vi "Parse Data Object Simple.vi"(11 "Data":T1(array[cluster])) -> (0 "ROI 1, Frame 1, Row 1":dbl[](graph), 3 "ROI 1, Frame 1":dbl[][](graph))   [LabVIEW 2015, in "LightField Automation.lvclass"]
uses:
  LightField Automation.lvclass
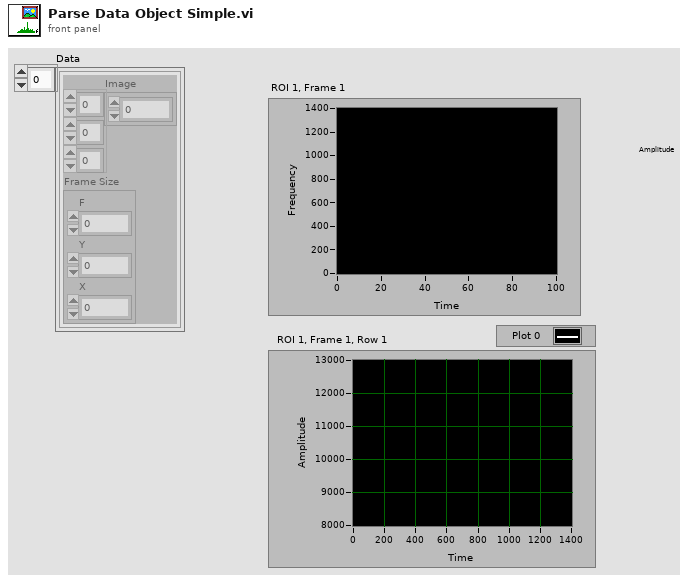
[diagram p1: front panel]
types:
  T1 = cluster{"Image":dbl[][][], "Frame Size":cluster{"F":i32, "Y":i32, "X":i32}}[]
  T2 = cluster{"Image":dbl[][][], "Frame Size":cluster{"F":i32, "Y":i32, "X":i32}}
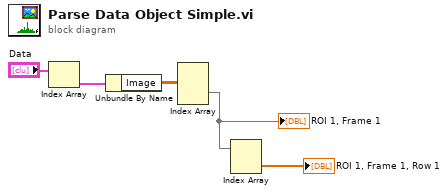
[diagram p0: block diagram]
diagram:
  n1 = Index Array(array="Data") -> (element=w5:T2)  [unwired: 1 in]
  n2 = Unbundle By Name(w5) -> ("Image"=w4:dbl[][][])
  n3 = Index Array(array=w4) -> (element=w3:dbl[][])  [unwired: 3 in]
  "ROI 1, Frame 1" <- w3
  n4 = Index Array(array=w3) -> (element=→"ROI 1, Frame 1, Row 1":dbl[])  [unwired: 2 in]
